vi "SysIdRoutine_Update.vi"(9 "MotorIO":T1, 11 "in SysIdRoutine":T4={"m_config"={"m_timeout_Sec"=10.0, "m_stepVoltage_Volt"=7.0, "m_rampRate_V/S"=1.0}, "m_mechanism"={"m_drive_volts"=0.0, "m_log"=[], "m_name"=""}, "m_outputVolts"=0.0, "m_recordState"=enum."kNone", "timer"={"StartTime"=0.0, "Accumulated TIme"=0.0, "Running"=FALSE, "semaphore"=refnum}} {"timer"."Accumulated TIme" format="%13.5p"; "timer"."StartTime" format="%13.5p"}) -> (3 "out SysIdRoutine":T4={"m_config"={"m_timeout_Sec"=10.0, "m_stepVoltage_Volt"=7.0, "m_rampRate_V/S"=1.0}, "m_mechanism"={"m_drive_volts"=0.0, "m_log"=[], "m_name"=""}, "m_outputVolts"=0.0, "m_recordState"=enum."kNone", "timer"={"StartTime"=0.0, "Accumulated TIme"=0.0, "Running"=FALSE, "semaphore"=refnum}} {"timer"."Accumulated TIme" format="%13.5p"; "timer"."StartTime" format="%13.5p"})   [LabVIEW 2023]
uses:
  <vilib>/Rock Robotics/WPI/ThirdParty/JAS_Junk/TrajLib/TypeDef/TIMER.ctl
  <vilib>/Utility/semaphor.llb/Obtain Semaphore Reference.vi
  <vilib>/Rock Robotics/WPI/ThirdParty/JAS_Junk/TrajLib/Timer_Reset.vi
  <vilib>/Rock Robotics/WPI/ThirdParty/JAS_Junk/TrajLib/Trajectory_Library.lvlib
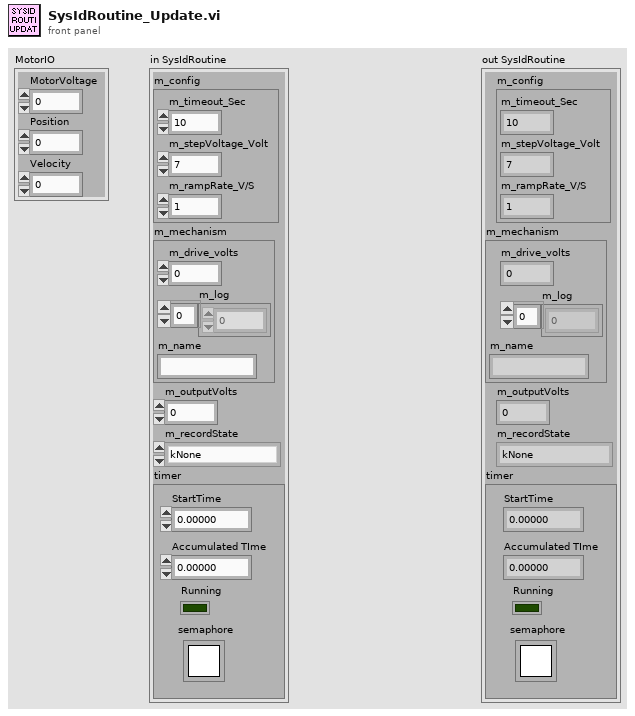
[diagram p1: front panel]
types:
  T1 = cluster{"MotorVoltage":dbl, "Position":dbl, "Velocity":dbl}
  T2 = typedef "Trajectory_Library.lvlib/TIMER.ctl" = cluster{"StartTime":dbl, "Accumulated TIme":dbl, "Running":bool, "semaphore":T3}
  T3 = typedef "Semaphore RefNum" = refnum<k1>
  T4 = cluster{"m_config":cluster{"m_timeout_Sec":dbl, "m_stepVoltage_Volt":dbl, "m_rampRate_V/S":dbl}, "m_mechanism":cluster{"m_drive_volts":dbl, "m_log":u8[], "m_name":string}, "m_outputVolts":dbl, "m_recordState":enum16{"kQuasistaticForward", "kQuasistaticReverse", "kDynamicForward", "kDynamicReverse", "kNone"}, "timer":T2}
  T5 = enum16{"big-endian, network order", "native, host order", "little-endian"}
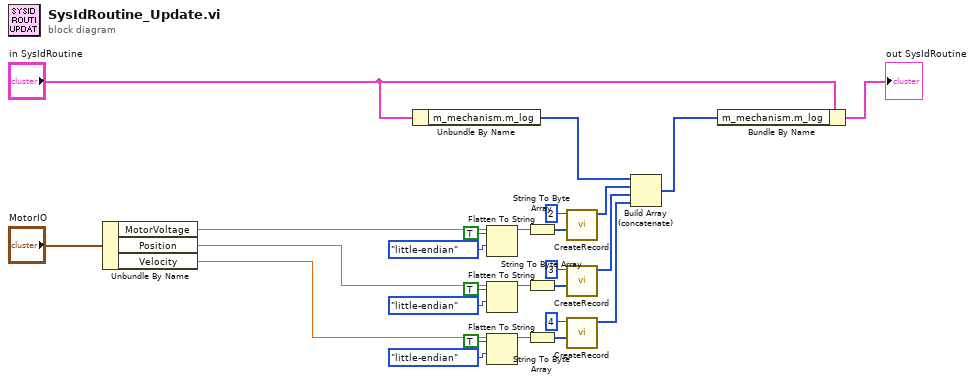
[diagram p0: block diagram]
diagram:
  n1 = Unbundle By Name("MotorIO") -> ("MotorVoltage"=w4:dbl, "Position"=w6:dbl, "Velocity"=w5:dbl)
  n2 = Unbundle By Name("in SysIdRoutine") -> ("m_mechanism.m_log"=w2:u8[])
  n3 = Flatten To String(anything=w4, prepend array or string size? (T)=TRUE, byte order (0:big-endian, network order)=T5."little-endian") -> (data string=w22:string)  [unwired: 1 in, 2 out]
  n4 = Flatten To String(anything=w6, prepend array or string size? (T)=TRUE, byte order (0:big-endian, network order)=T5."little-endian") -> (data string=w17:string)  [unwired: 1 in, 2 out]
  n5 = Flatten To String(anything=w5, prepend array or string size? (T)=TRUE, byte order (0:big-endian, network order)=T5."little-endian") -> (data string=w12:string)  [unwired: 1 in, 2 out]
  n6 = String To Byte Array(string=w22) -> (unsigned byte array=w23:u8[])
  n7 = String To Byte Array(string=w17) -> (unsigned byte array=w16:u8[])
  n8 = String To Byte Array(string=w12) -> (unsigned byte array=w13:u8[])
  n9 = call "CreateRecord.vi"("payload data (little endian)"=w23, "entry ID"=2) -> ("record"=w9:u8[])  [unwired: 9 in]
  n10 = call "CreateRecord.vi"("payload data (little endian)"=w16, "entry ID"=3) -> ("record"=w8:u8[])  [unwired: 9 in]
  n11 = call "CreateRecord.vi"("payload data (little endian)"=w13, "entry ID"=4) -> ("record"=w7:u8[])  [unwired: 9 in]
  n12 = Build Array (concatenate)(w2, w9, w8, w7) -> (w3:u8[])
  n13 = Bundle By Name(cluster="in SysIdRoutine", "m_mechanism.m_log"=w3) -> (→"out SysIdRoutine":T4)
